vi "Write filter.vi"(8 "error in":errorcluster, 10 "filter":bool, 11 "CRDS Data in":refnum<class "CRDS Data.lvclass">) -> (0 "error out":errorcluster, 3 "CRDS Data out":refnum<class "CRDS Data.lvclass">)   [LabVIEW 2015, in "CRDS Data.lvclass"]
uses:
  CRDS Data.lvclass
  CRDS Data.lvclass/CRDS Data.ctl
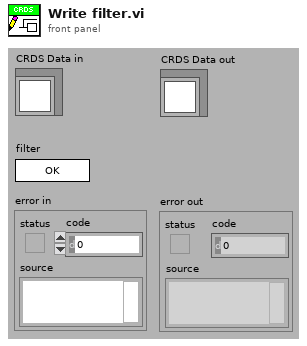
[diagram p1: front panel]
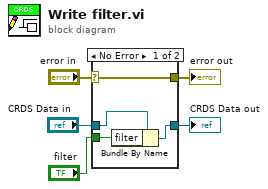
[diagram p0: block diagram]
diagram:
  n1 = case shown="No Error" "error in" {
    selector: "error in" -> [w9 w10]
    tunnel: [w9 w10] -> w4
    tunnel: [w7 w11] -> w2
    tunnel: "CRDS Data in" -> [w8 w11]
    tunnel: "filter" -> [w6 _]
    frame No Error {
      n2 = Bundle By Name(cluster=w8, "filter"=w6) -> (w7:refnum<class "CRDS Data.lvclass">)
    }
    frame Error {
    }
  }
  "error out" <- w4
  "CRDS Data out" <- w2
